vi "Exit.vi"(8 "error in (no error)":errorcluster, 11 "Old State":refnum<class "Guide.lvclass">) -> (0 "error out":errorcluster, 3 "New State":refnum<class "Guide.lvclass">)   [LabVIEW 2014, in "States.lvlib" / "Guide.lvclass"]
doc: "This is an abstract method. Override this method to define the behavior when you leave the state."
uses:
  Guide.lvclass
  <vilib>/ActorFramework/Message Enqueuer/Message Enqueuer.lvclass/Message Enqueuer.ctl
  <vilib>/ActorFramework/Message Enqueuer/Enqueue.vi
  <vilib>/ActorFramework/Message Priority Queue/Priority Enqueue.vi
  Global_var/Global_var.vi
  Process State/CoordinatorState.lvclass
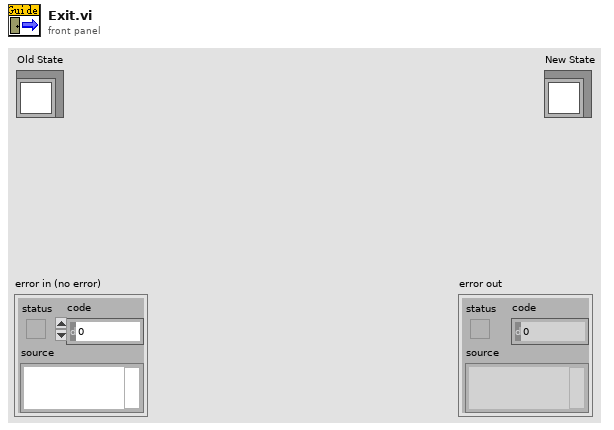
[diagram p1: front panel]
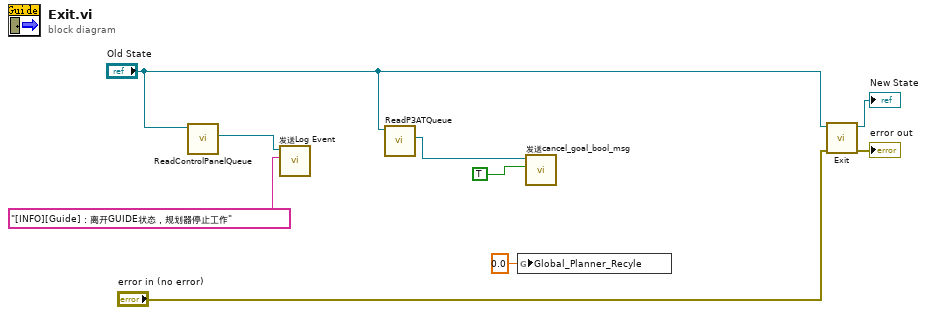
[diagram p0: block diagram]
diagram:
  n1 = call-dynamic "ReadControlPanelQueue.vi"("CoordinatorState输入"="Old State") -> ("操作者框架:消息待入队列"=w6:refnum<class "Message Enqueuer.lvclass">)  [unwired: 8 in, 2 out]
  n2 = call "发送Log Event.vi"("Event Text"="[INFO][Guide]：离开GUIDE状态，规划器停止工作", "消息待入队列"=w6) -> ()  [unwired: 8 in, 2 out]
  n3 = call-dynamic "ReadP3ATQueue.vi"("CoordinatorState输入"="Old State") -> ("操作者框架:消息待入队列"=w4:refnum<class "Message Enqueuer.lvclass">)  [unwired: 8 in, 2 out]
  n4 = global write "Global_var.vi" "Global_Planner_Recyle"(0.0 ("Global_Planner_Recyle")) -> ()
  n5 = call "发送cancel_goal_bool_msg.vi"("值(信号)"=TRUE, "消息待入队列"=w4) -> ()  [unwired: 8 in, 2 out]
  n6 = call-parent "Exit.vi"("error in (no error)"="error in (no error)", "Old State"="Old State") -> ("error out"=→"error out":errorcluster, "New State"=→"New State":refnum<class "Guide.lvclass">)  [unwired: 8 in]
